vi "Stop Core.vi"(10 "final error code":i32 caption="最终错误代码", 11 "客户端代理者 in":refnum<class "客户端代理者.lvclass"> caption="操作者输入") -> (3 "客户端代理者 out":refnum<class "客户端代理者.lvclass"> caption="操作者输出")   [LabVIEW 2015, in "客户端代理者.lvlib" / "客户端代理者.lvclass"]
doc: "(<B>文件名</B>: Actor Framework.lvlib:Actor.lvclass:Stop Core.vi)\n\n定义停止前操作者的动作。Use the <B>final error code</B> input to determine whether the actor shut down in response to an error.\n\nBy default, this method passes the Stop message along to all auto-stop nested actors.A descendant class may override this method to define additional behavior, such as shutting down any processes the actor initiated in its override of the Actor Core method."
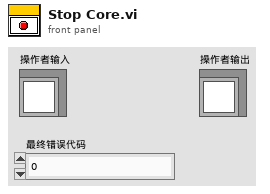
[diagram p1: front panel]
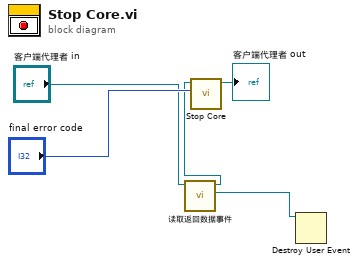
[diagram p0: block diagram]
diagram:
  n1 = call-dynamic "读取返回数据事件.vi"("通讯输入"="客户端代理者 in") -> ("返回数据事件"=w2:refnum<user-event>, "通讯输出"=w1:refnum<class "客户端代理者.lvclass">)  [unwired: 8 in, 1 out]
  n2 = call-parent "Stop Core.vi"("final error code"="final error code", "通讯 in"=w1) -> ("通讯 out"=→"客户端代理者 out":refnum<class "客户端代理者.lvclass">)  [unwired: 9 in]
  n3 = Destroy User Event(user event=w2) -> ()  [unwired: 1 in, 1 out]
